vi "[W] Generic Watchdog.vi"() -> ()   [LabVIEW 2014]
uses:
  Sensor Reading.ctl
  <vilib>/NI/Tools/String/Tools_String.lvlib
panel:
  in  "Message Q":refnum<queue>
  in  "Data Q":refnum<queue>
  in  "Sensor Reading":T1
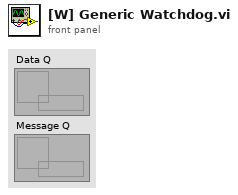
[diagram p1: front panel]
types:
  T1 = typedef "Sensor Reading.ctl" = cluster{"Sensor Name":string, "Timestamp":string, "Data Chunk":string}
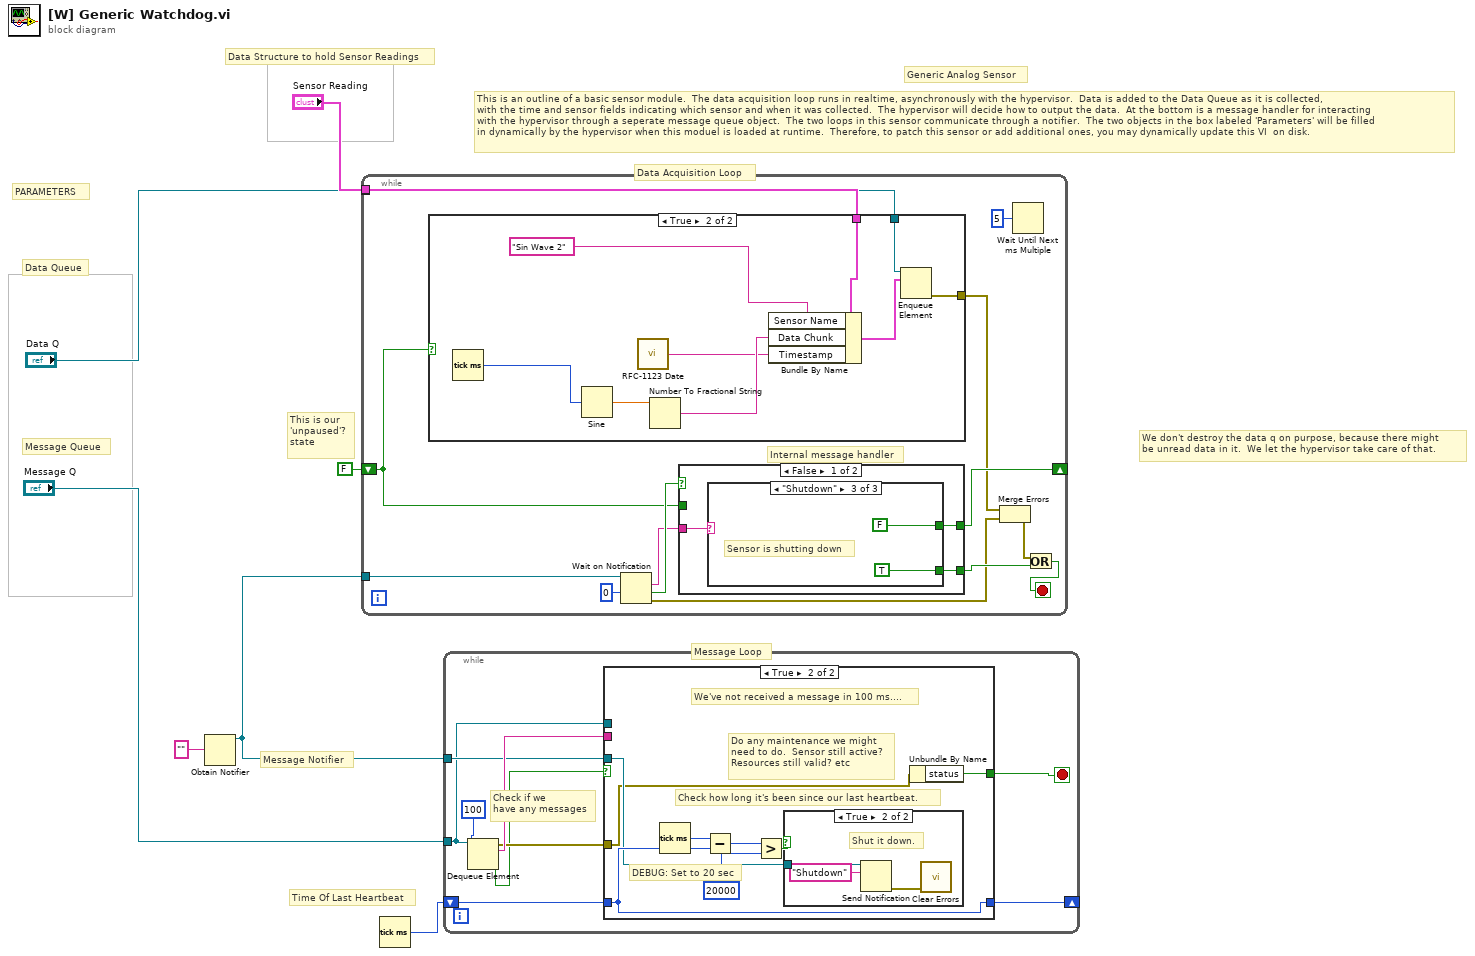
[diagram p0: block diagram]
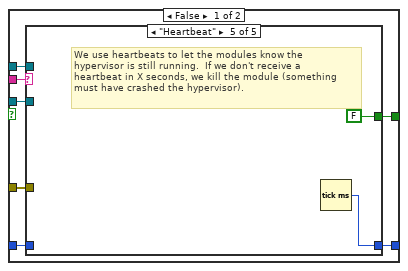
[diagram p2: hidden frame]
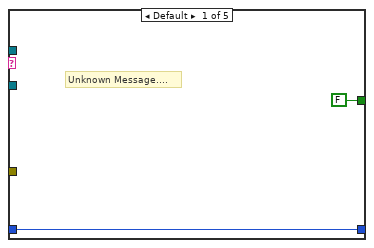
[diagram p3: hidden frame]
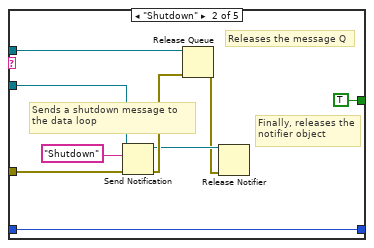
[diagram p4: hidden frame]
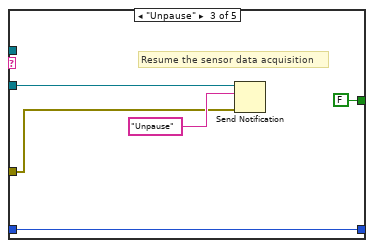
[diagram p5: hidden frame]
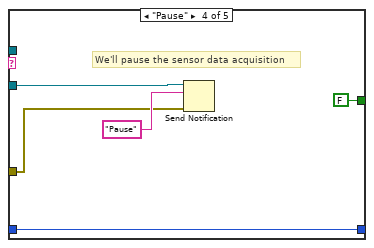
[diagram p6: hidden frame]
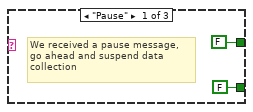
[diagram p9: hidden frame]
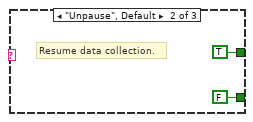
[diagram p10: hidden frame]
diagram:
  # "Time Of Last Heartbeat"
  # "This is an outline of a basic sensor module.  The data acquisition loop runs in realtime, asynchronously with the hypervisor.  Data is added to the Data Queue as it is collected,\nwith the time and sensor fields indicating which sensor and when it was collected.  The hypervisor will decide how to output the data.  At the bottom is a message handler for interacting\nwith the hypervisor through a seperate message queue object.  The two loops in this sensor communicate through a notifier.  The two objects in the box labeled 'Parameters' will be filled\nin dynamically by the hypervisor when this moduel is loaded at runtime.  Therefore, to patch this sensor or add additional ones, you may dynamically update this VI  on disk."
  # "This is our\n'unpaused'?\nstate"
  # "We don't destroy the data q on purpose, because there might\nbe unread data in it.  We let the hypervisor take care of that."
  # "Data Structure to hold Sensor Readings"
  # "Data Acquisition Loop"
  # "Message Loop"
  # "Message Notifier"
  # "Message Queue"
  # "Data Queue"
  # "PARAMETERS"
  # "Generic Analog Sensor"
  n1 = Obtain Notifier(notification data type="") -> (notifier out=w1:refnum<notifier>)  [unwired: 3 in, 2 out]
  n2 = while {
    tunnel: "Data Q" -> [w12]
    tunnel: "Sensor Reading" -> [w19]
    tunnel: w1 -> [w21]
    shift-right: [w16] -> _
    shift-left: FALSE -> [w15]
    stop <- w11 stop-if-true
    # "Internal message handler"
    n3 = case shown="True" w15 {
      tunnel: w12 -> [_ w28]
      tunnel: w19 -> [_ w23]
      tunnel: [_ w24] -> w10
      frame False {
      }
      frame True {
        n4 = Tick Count (ms)() -> (millisecond timer value=w30:u32)
        n5 = Sine(x=w30) -> (sin(x)=w29:dbl)
        n6 = call <vilib>:"RFC-1123 Date.vi"() -> ("GMT Date/Time"=w22:string)  [unwired: 2 in]
        n7 = Number To Fractional String(number=w29) -> (F-format string=w27:string)  [unwired: 3 in]
        n8 = Bundle By Name(cluster=w23, "Sensor Name"="Sin Wave 2", "Data Chunk"=w27, "Timestamp"=w22) -> (w25:T1)
        n9 = Enqueue Element(queue=w28, element=w25) -> (error out=w24:errorcluster)  [unwired: 2 in, 2 out]
      }
    }
    n10 = Wait on Notification(notifier=w21, timeout in ms (-1)=0) -> (notification=w17:string, timed out?=w18:bool, error out=w9:errorcluster)  [unwired: 2 in, 1 out]
    n11 = case shown="False" w18 {
      tunnel: w17 -> [w33 _]
      tunnel: [w32 _] -> w14
      tunnel: [w31 w40] -> w16
      tunnel: w15 -> [_ w40]
      frame False {
        n12 = case shown="\"Shutdown\"" w33 {
          tunnel: [FALSE FALSE TRUE] -> w32
          tunnel: [FALSE TRUE FALSE] -> w31
          frame "Pause" {
            # "We received a pause message,\ngo ahead and suspend data collection"
          }
          frame "Unpause", Default {
            # "Resume data collection."
          }
          frame "Shutdown" {
            # "Sensor is shutting down"
          }
        }
      }
      frame True {
      }
    }
    n13 = Merge Errors(w10, w9) -> (w8:errorcluster)
    n14 = Wait Until Next ms Multiple(millisecond multiple=u32 5) -> ()  [unwired: 1 out]
    n15 = Or(x=w8, y=w14) -> (x .or. y?=w11:bool)
  }
  n16 = Tick Count (ms)() -> (millisecond timer value=w2:u32)
  n17 = while {
    tunnel: "Message Q" -> [w46]
    tunnel: w1 -> [w47]
    shift-right: [w41] -> _
    shift-left: w2 -> [w42]
    stop <- w48 stop-if-true
    # "Check if we \nhave any messages"
    n18 = Dequeue Element(queue=w46, timeout in ms (-1)=100) -> (element=w49:string, timed out?=w43:bool, error out=w45:errorcluster)  [unwired: 1 in, 1 out]
    n19 = case shown="True" w43 {
      tunnel: w49 -> [w56 _]
      tunnel: [w55 w80] -> w48
      tunnel: w47 -> [w54 w82]
      tunnel: w46 -> [w53 _]
      tunnel: w45 -> [w52 w81]
      tunnel: w42 -> [w51 w83]
      tunnel: [w50 w83] -> w41
      frame False {
        n20 = case shown="\"Heartbeat\"" w56 {
          tunnel: [FALSE TRUE FALSE FALSE FALSE] -> w55
          tunnel: w54 -> [_ w65 w70 w74 _]
          tunnel: w53 -> [_ w66 _ _ _]
          tunnel: w52 -> [_ w64 w71 w75 _]
          tunnel: w51 -> [w57 w59 w68 w73 _]
          tunnel: [w57 w59 w68 w73 w79] -> w50
          frame Default {
            # "Unknown Message...."
          }
          frame "Shutdown" {
            # "Finally, releases the\nnotifier object"
            # "Releases the message Q"
            # "Sends a shutdown message to \nthe data loop"
            n21 = Send Notification(notification="Shutdown", notifier=w65, error in (no error)=w64) -> (notifier out=w61:refnum<notifier>, error out=w63:errorcluster)
            n22 = Release Queue(queue=w66, error in (no error)=w63) -> (error out=w60:errorcluster)  [unwired: 1 in, 2 out]
            n23 = Release Notifier(notifier=w61, error in (no error)=w60) -> ()  [unwired: 1 in, 3 out]
          }
          frame "Unpause" {
            # "Resume the sensor data acquisition"
            n24 = Send Notification(notification="Unpause", notifier=w70, error in (no error)=w71) -> ()  [unwired: 2 out]
          }
          frame "Pause" {
            # "We'll pause the sensor data acquisition"
            n25 = Send Notification(notification="Pause", notifier=w74, error in (no error)=w75) -> ()  [unwired: 2 out]
          }
          frame "Heartbeat" {
            # "We use heartbeats to let the modules know the \nhypervisor is still running.  If we don't receive a\nheartbeat in X seconds, we kill the module (something\nmust have crashed the hypervisor)."
            n26 = Tick Count (ms)() -> (millisecond timer value=w79:u32)
          }
        }
      }
      frame True {
        # "DEBUG: Set to 20 sec"
        # "Check how long it's been since our last heartbeat."
        # "Do any maintenance we might\nneed to do.  Sensor still active?\nResources still valid? etc"
        # "We've not received a message in 100 ms...."
        n27 = Tick Count (ms)() -> (millisecond timer value=w87:u32)
        n28 = Subtract(x=w87, y=w83) -> (x-y=w86:u32)
        n29 = Greater?(x=w86, y=u32 20000) -> (0:w84:bool)
        n30 = case shown="True" w84 {
          tunnel: w82 -> [_ w90]
          frame False {
          }
          frame True {
            # "Shut it down."
            n31 = Send Notification(notification="Shutdown", notifier=w90) -> (error out=w88:errorcluster)  [unwired: 1 in, 1 out]
            n32 = call <vilib>:"Clear Errors.vi"("error in (no error)"=w88) -> ()  [unwired: 5 in, 2 out]
          }
        }
        n33 = Unbundle By Name(w81) -> ("status"=w80:bool)
      }
    }
  }
